vi "Interpolate Y (single).vi"(8 "error in (no error)":errorcluster, 10 "x (0)":dbl, 11 "XY-data":cluster{"X-array":dbl[], "Y-array":dbl[]}) -> (0 "error out":errorcluster, 2 "y":dbl, 3 "XY-data out":cluster{"X-array":dbl[], "Y-array":dbl[]} {"Y-array" format="%.2p"; "X-array" format="%.2p"})   [LabVIEW 2016, in "xy_utilities.lvlib"]
doc: "Shift the zero value of the x array by giving a new fractional x index.\n\nWire data to the data input to determine the polymorphic instance to use or manually select the instance."
uses:
  xy_utilities.lvlib
  Sort (single).vi
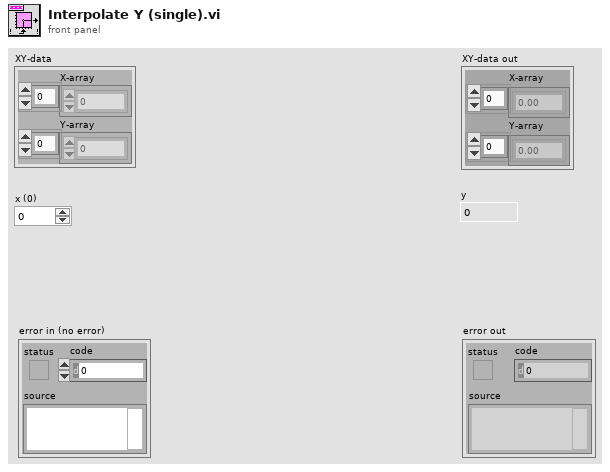
[diagram p1: front panel]
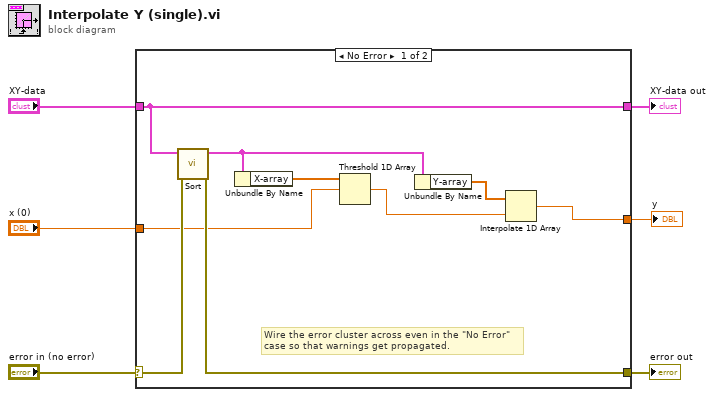
[diagram p0: block diagram]
diagram:
  n1 = case shown="No Error" "error in (no error)" {
    selector: "error in (no error)" -> [w14 w17]
    tunnel: [w13 w17] -> w5
    tunnel: "XY-data" -> [w15 w16]
    tunnel: [w15 w16] -> w3
    tunnel: "x (0)" -> [w10 _]
    tunnel: [w9 _] -> w1
    frame No Error {
      # "Wire the error cluster across even in the \"No Error\"\ncase so that warnings get propagated."
      n2 = call-poly "Sort.vi"("error in (no error)"=w14, "XY-data"=w15) -> ("error out"=w13:errorcluster, "Sorted XY-data out"=w11:cluster{"X-array":dbl[], "Y-array":dbl[]})  [unwired: 8 in]
      n3 = Unbundle By Name(w11) -> ("X-array"=w12:dbl[])
      n4 = Threshold 1D Array(2:w10, 3:w12) -> (0:w7:dbl)  [unwired: 1 in]
      n5 = Unbundle By Name(w11) -> ("Y-array"=w8:dbl[])
      n6 = Interpolate 1D Array(1:w7, 2:w8) -> (0:w9:dbl)
    }
    frame Error {
    }
  }
  "error out" <- w5
  "XY-data out" <- w3
  "y" <- w1
